vi "IO Enable.vi"(8 "error in (no error)":errorcluster, 10 "enable":u8, 11 "channel":u8) -> (0 "error out":errorcluster)   [LabVIEW 2021, in "vmmso.lvlib"]
doc: "DLL_API void WINAPI IOEnable(unsigned char channel, unsigned char enable);"
uses:
  vmmso.lvlib
  vmmso.dll
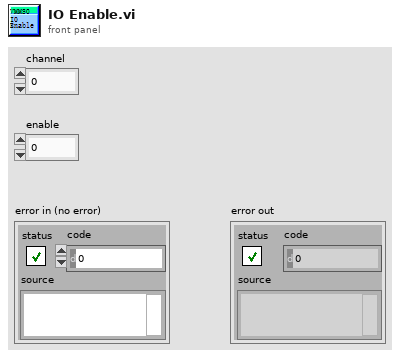
[diagram p1: front panel]
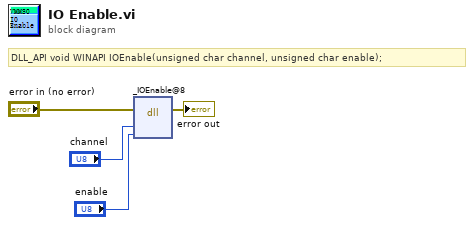
[diagram p0: block diagram]
diagram:
  # "DLL_API void WINAPI IOEnable(unsigned char channel, unsigned char enable);"
  n1 = dll-call lib="O:/MSO/library/demo-Labview/vmmso/vmmso.*" fn="_IOEnable@8"(error in="error in (no error)", "channel"="channel", "enable"="enable") -> (error out=→"error out":errorcluster)  [unwired: 5 in, 1 out]
